vi "Send_Get_1Bit.vi"(8 "error in (no error)":errorcluster, 10 "Channel":u8, 11 "Simulated uC in":refnum<class "Simulated uC.lvclass">) -> (0 "error out":errorcluster, 2 "buffer":string, 3 "Simulated uC out":refnum<class "Simulated uC.lvclass">)   [LabVIEW 2019, in "Simulated uC.lvclass"]
uses:
  Simulated uC.lvclass
  Clase Padre/Serial Device.lvclass
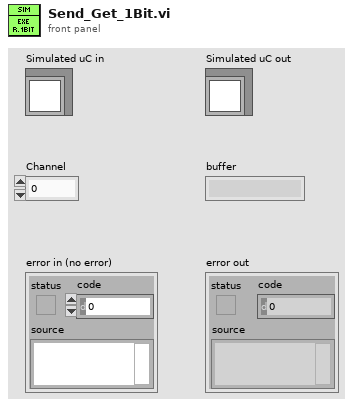
[diagram p1: front panel]
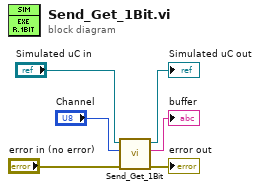
[diagram p0: block diagram]
diagram:
  n1 = call-parent "Send_Get_1Bit.vi"("error in (no error)"="error in (no error)", "Channel"="Channel", "Serial Device in"="Simulated uC in") -> ("error out"=→"error out":errorcluster, "buffer"=→"buffer":string, "Serial Device out"=→"Simulated uC out":refnum<class "Simulated uC.lvclass">)  [unwired: 6 in]
